vi "Scale Settings Dialog.vi"(8 "error in (no error)":errorcluster, 11 "Scale Module Config In":T1={"GUID"="", "Drop Coords"={"Horizontal"=0, "Vertical"=0}, "Process Name"="", "User name"="", "Queue Name"="", "Settings"={"Cycle Period"=500.0, "Mettler"={"VISA resource name"="", "Simulated?"=FALSE}, "Scale Type"=""}, "Load Count"=0}) -> (0 "error out":errorcluster, 1 "Cancelled?":bool=TRUE, 2 "UI Refresh Needed?":bool, 3 "Scale Module Config Out":T1={"GUID"="", "Drop Coords"={"Horizontal"=0, "Vertical"=0}, "Process Name"="", "User name"="", "Queue Name"="", "Settings"={"Cycle Period"=500.0, "Mettler"={"VISA resource name"="", "Simulated?"=FALSE}, "Scale Type"=""}, "Load Count"=0})   [LabVIEW 2018, in "Scale Module.lvlib"]
doc: "Dialog for selecting user specified settings."
uses:
  Scale Module.lvlib
  Feed Module/Controls/Scale Module Settings Cluster.ctl
  Mettler Toledo/Controls/Settings Cluster.ctl
  Feed Module/Controls/Scale Module Config Cluster.ctl
  <vilib>/Utility/miscctls.llb/LVPoint32TypeDef.ctl
  <vilib>/Utility/xml.llb/Write to XML File(string).vi
  Settings/Settings.lvlib
  Mettler Toledo/Mettler Toledo.lvlib
panel:
  in  "Module Name":string
  in  "Scale Configurations":T3={"Cycle Period"=500.0, "Mettler"={"VISA resource name"="", "Simulated?"=FALSE}, "Scale Type"="Default"}
  in  "Cancel Button":bool
  in  "OK Button":bool
  # "Non visible portion of dialog (needed for connector pane)."
  # "Scale Settings"
  # "Scale Settings"
  # "Scale Settings"
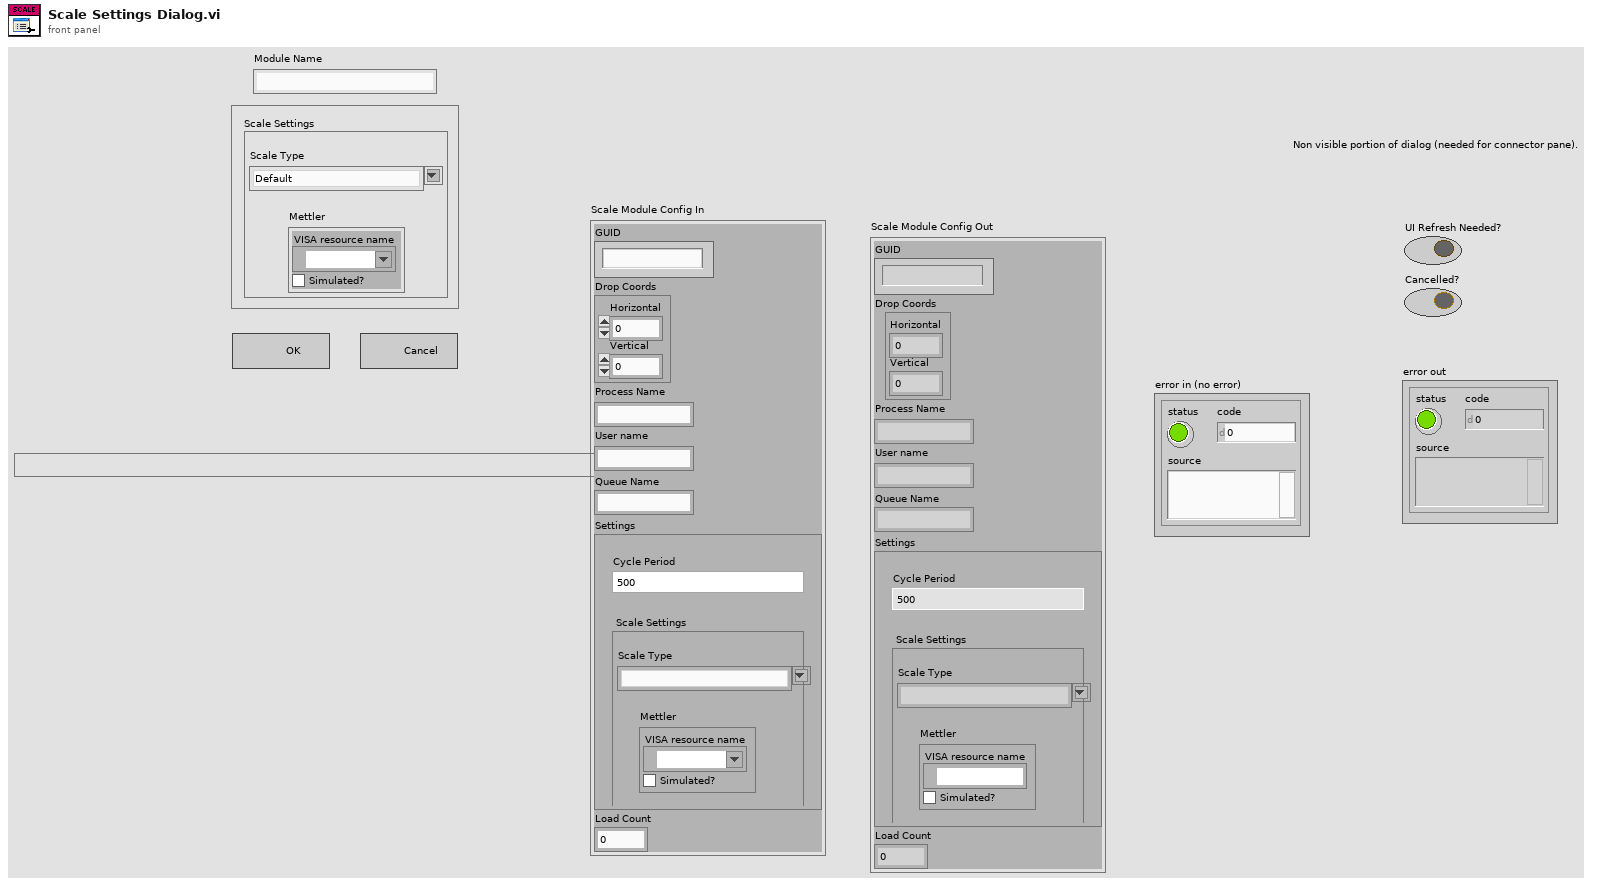
[diagram p1: front panel]
types:
  T1 = typedef "Scale Module.lvlib/Scale Module Config Cluster.ctl" = cluster{"GUID":string, "Drop Coords":T2, "Process Name":string, "User name":string, "Queue Name":string, "Settings":T3, "Load Count":i32}
  T2 = typedef "LVPoint32TypeDef.ctl" = cluster{"Horizontal":i32, "Vertical":i32}
  T3 = typedef "Scale Module.lvlib/Scale Module Settings Cluster.ctl" = cluster{"Cycle Period":dbl, "Mettler":T4, "Scale Type":string}
  T4 = typedef "Mettler Toledo.lvlib/Settings Cluster.ctl" = cluster{"VISA resource name":refnum<visa-resource-name>, "Simulated?":bool}
  T5 = enum8{"Enabled", "Disabled", "Disabled and Grayed Out"}
  T6 = cluster{"Cycle Period":dbl, "Mettler":T4, "Scale Type":string}
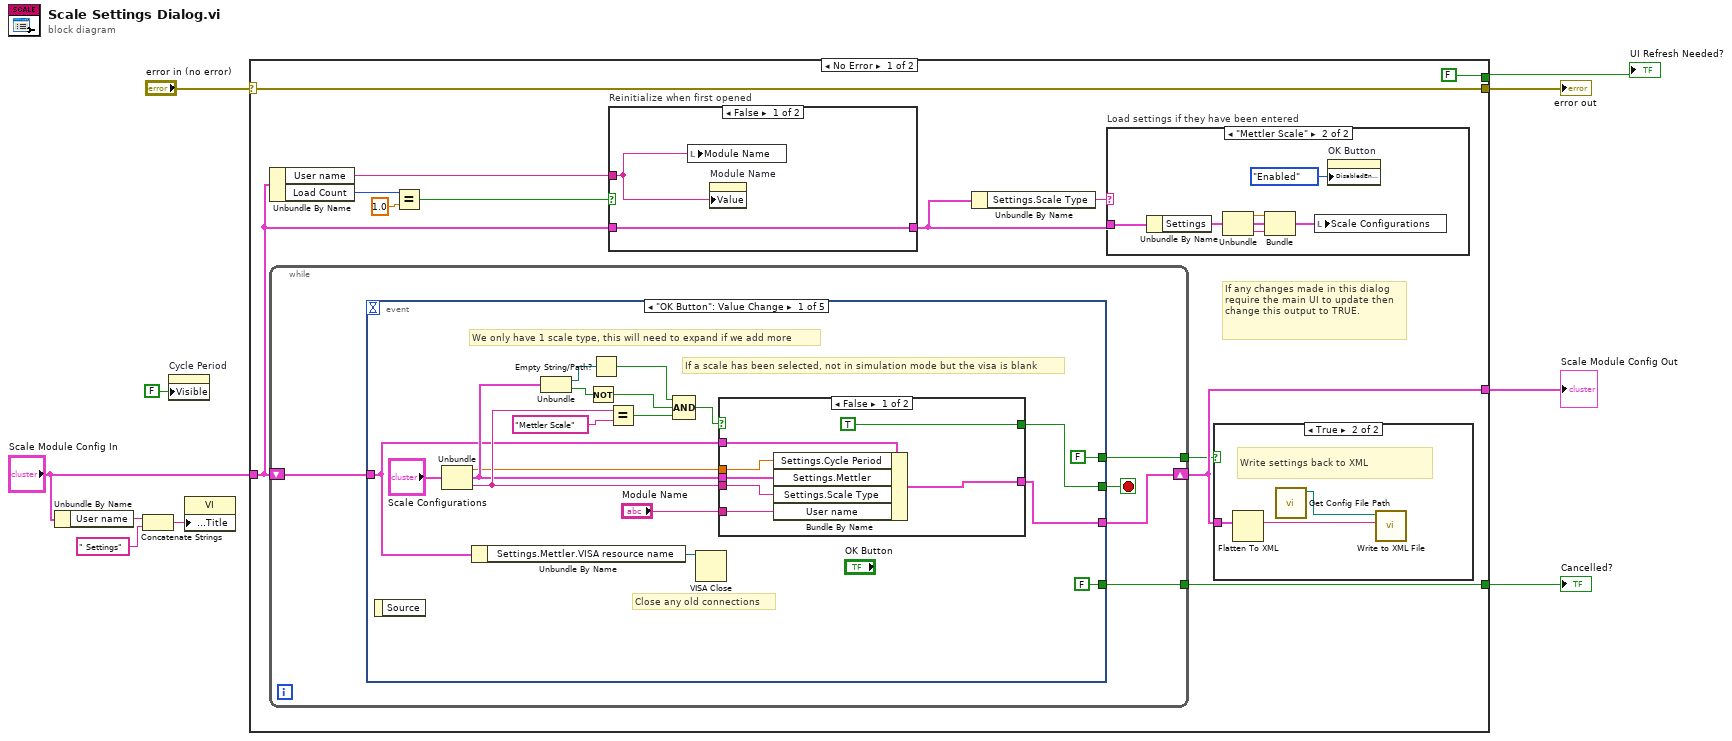
[diagram p0: block diagram]
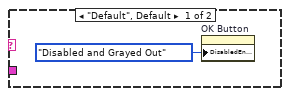
[diagram p2: hidden frame]
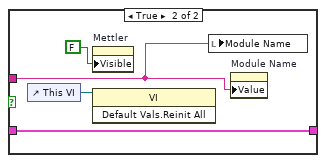
[diagram p3: hidden frame]
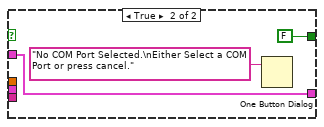
[diagram p4: hidden frame]
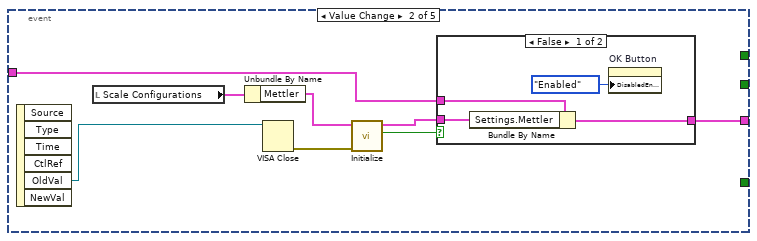
[diagram p5: hidden frame]
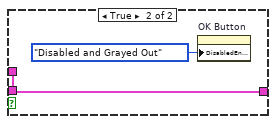
[diagram p6: hidden frame]
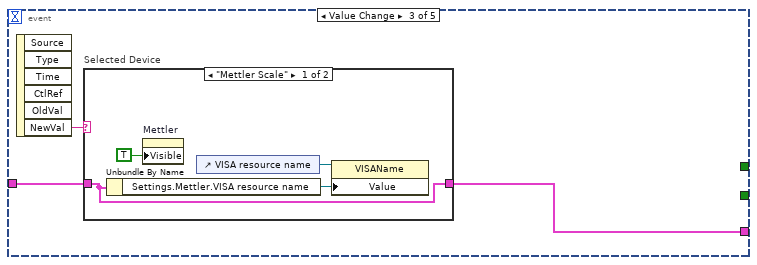
[diagram p7: hidden frame]
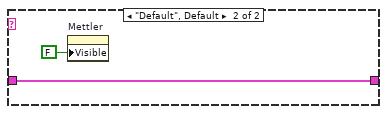
[diagram p8: hidden frame]
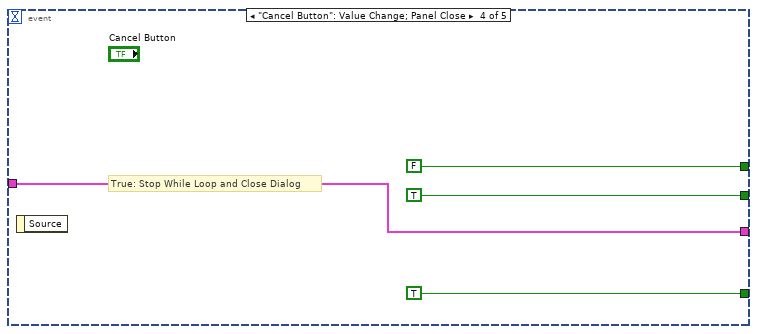
[diagram p9: hidden frame]
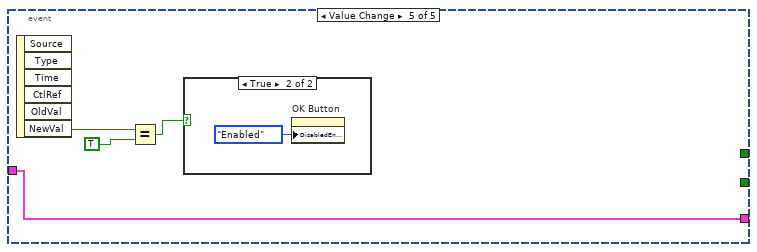
[diagram p10: hidden frame]
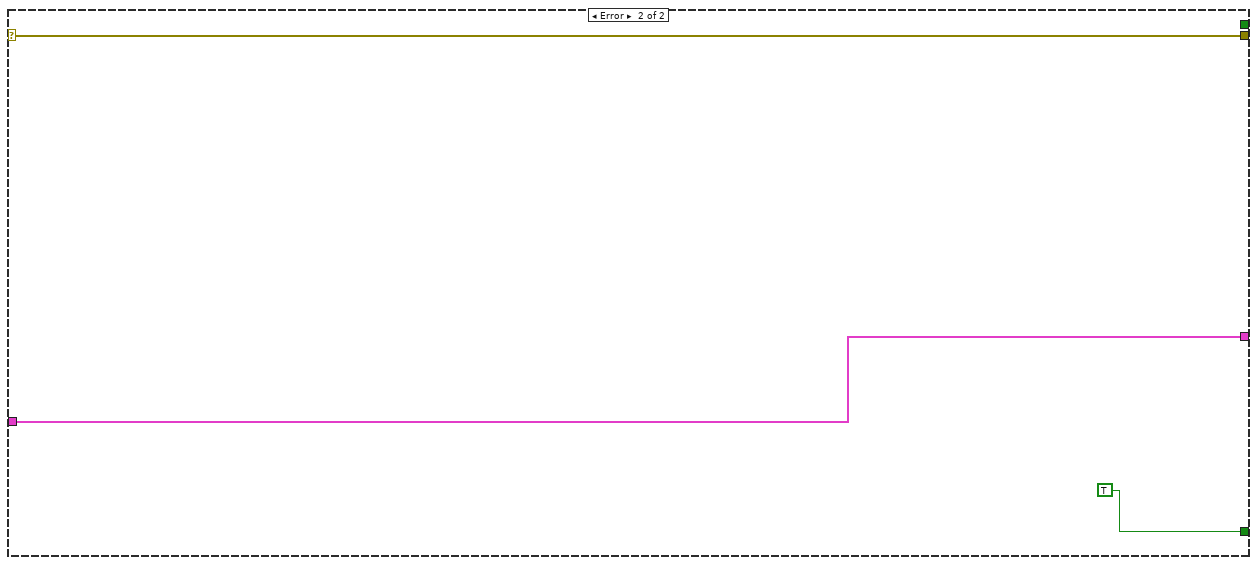
[diagram p13: hidden frame]
diagram:
  n1 = Unbundle By Name("Scale Module Config In") -> ("User name"=w1:string)
  n2 = Concatenate Strings(w1, " Settings" ("string")) -> (w4:string)
  n3 = property on="Cycle Period" class="DigNum (strict)"("Visible"=FALSE) -> ()  [unwired: 2 in, 2 out]
  n4 = property class="VI"("Front Panel.Title"=w4) -> ()  [unwired: 2 in, 2 out]
  n5 = case shown="No Error" "error in (no error)" {
    selector: "error in (no error)" -> [w22 w107]
    tunnel: [w22 w107] -> w10
    tunnel: "Scale Module Config In" -> [w12 w106]
    tunnel: [w20 w106] -> w6
    tunnel: [FALSE ("UI Refresh Needed?") _] -> w9
    tunnel: [w16 TRUE ("UI Refresh Needed?")] -> w8
    frame No Error {
      # "If any changes made in this dialog require the main UI to update then change this output to TRUE."
      n6 = Unbundle By Name(w12) -> ("User name"=w11:string, "Load Count"=w19:i32)
      n7 = while {
        tunnel: [w41] -> w17
        tunnel: [w38] -> w16
        shift-right: [w40] -> w20
        shift-left: w12 -> [w37]
        stop <- w39 stop-if-true
        n8 = event shown="[0] \"OK Button\": Value Change" {
          selector: _ -> [_ _ _ _ _]
          dyn-events: _ -> [_ _ _ _ _]
          timeout: _ -> [_ _ _ _ _]
          tunnel: [w57 w75 w85 w96 w100] -> w40
          tunnel: w37 -> [w48 w76 w84 w96 w100]
          tunnel: [FALSE ("UI Refresh Needed?") _ _ FALSE ("UI Refresh Needed?") _] -> w41
          tunnel: [w58 _ _ TRUE _] -> w39
          tunnel: [FALSE ("UI Refresh Needed?") _ _ TRUE ("UI Refresh Needed?") _] -> w38
          event "OK Button": Value Change {
            # "Close any old connections"
            # "If a scale has been selected, not in simulation mode but the visa is blank"
            # "We only have 1 scale type, this will need to expand if we add more"
            n9 = event-data() -> ()  [unwired: 1 in, 1 out]
            n10 = Unbundle("Scale Configurations") -> ("Cycle Period"=w51:dbl, "Mettler"=w52:T4, "Scale Type"=w54:string)
            n11 = Unbundle By Name(w48) -> ("Settings.Mettler.VISA resource name"=w47:refnum<visa-resource-name>)
            n12 = Unbundle(w52) -> ("VISA resource name"=w55:refnum<visa-resource-name>, "Simulated?"=w50:bool)
            n13 = Not(x=w50) -> (.not. x?=w44:bool)
            n14 = Empty String/Path?(string/path=w55) -> (empty?=w45:bool)
            n15 = Equal?(x=w54, y="Mettler Scale") -> (x = y?=w43:bool)
            n16 = Compound Arithmetic op=AND(w45, w44, w43) -> (w42:bool)
            n17 = VISA Close(VISA resource name=w47) -> ()  [unwired: 1 in, 1 out]
            n18 = case shown="False" w42 {
              tunnel: [TRUE FALSE] -> w58
              tunnel: [w65 w68] -> w57
              tunnel: w48 -> [w64 w68]
              tunnel: w54 -> [w63 _]
              tunnel: w52 -> [w62 _]
              tunnel: w51 -> [w61 _]
              tunnel: "Module Name" -> [w60 _]
              frame False {
                n19 = Bundle By Name(cluster=w64, "Settings.Cycle Period"=w61, "Settings.Mettler"=w62, "Settings.Scale Type"=w63, "User name"=w60) -> (w65:T1)
              }
              frame True {
                n20 = One Button Dialog(message="No COM Port Selected.\nEither Select a COM Port or press cancel.") -> ()  [unwired: 1 in, 1 out]
              }
            }
          }
          event Value Change {
            n21 = event-data() -> ("OldVal"=w71:refnum<visa-resource-name>)  [unwired: 1 in, 5 out]
            n22 = local read "Scale Configurations"() -> (w77:T3)
            n23 = Unbundle By Name(w77) -> ("Mettler"=w74:T4)
            n24 = VISA Close(VISA resource name=w71) -> (error out=w72:errorcluster)  [unwired: 1 in]
            n25 = call "Initialize.vi"("error in (no error)"=w72, "Mettler Settings in"=w74) -> ("No Scale Connected"=w70:bool, "Mettler Settings out"=w73:T4)  [unwired: 7 in, 1 out]
            n26 = case shown="False" w70 {
              tunnel: w76 -> [w81 w83]
              tunnel: [w80 w83] -> w75
              tunnel: w73 -> [w79 _]
              frame False {
                n27 = Bundle By Name(cluster=w81, "Settings.Mettler"=w79) -> (w80:T1)
                n28 = property on="OK Button" class="Bool"("DisabledEnum"=T5."Enabled" ("Disabled")) -> ()  [unwired: 2 in, 2 out]
              }
              frame True {
                n29 = property on="OK Button" class="Bool"("DisabledEnum"=T5."Disabled and Grayed Out" ("Disabled")) -> ()  [unwired: 2 in, 2 out]
              }
            }
          }
          event Value Change {
            n30 = event-data() -> ("NewVal"=w86:string)  [unwired: 1 in, 5 out]
            n31 = case "Selected Device" shown="\"Mettler Scale\"" w86 {
              tunnel: [w87 w92] -> w85
              tunnel: w84 -> [w87 w92]
              frame "Mettler Scale" {
                n32 = Unbundle By Name(w87) -> ("Settings.Mettler.VISA resource name"=w90:refnum<visa-resource-name>)
                n33 = property on="Mettler" class="Clust (strict)"("Visible"=TRUE) -> ()  [unwired: 2 in, 2 out]
                n34 = control-ref of="VISA resource name"() -> (w88:refnum<vi>)
                n35 = property on="Property Node" class="VISAName"(reference=w88, "Value"=w90) -> ()  [unwired: 1 in, 2 out]
              }
              frame "Default", Default {
                n36 = property on="Mettler" class="Clust (strict)"("Visible"=FALSE) -> ()  [unwired: 2 in, 2 out]
              }
            }
          }
          event "Cancel Button": Value Change; Panel Close {
            # "True: Stop While Loop and Close Dialog"
            n37 = event-data() -> ()  [unwired: 1 in, 1 out]
          }
          event Value Change {
            n38 = event-data() -> ("NewVal"=w98:bool)  [unwired: 1 in, 5 out]
            n39 = Equal?(x=w98, y=TRUE) -> (x = y?=w97:bool)
            n40 = case shown="True" w97 {
              frame False {
              }
              frame True {
                n41 = property on="OK Button" class="Bool"("DisabledEnum"=T5."Enabled" ("Disabled")) -> ()  [unwired: 2 in, 2 out]
              }
            }
          }
        }
      }
      n42 = Equal?(x=w19, y=1.0) -> (x = y?=w15:bool)
      n43 = case "Reinitialize when first opened" shown="False" w15 {
        tunnel: w12 -> [w32 w35]
        tunnel: [w32 w35] -> w13
        tunnel: w11 -> [w31 w33]
        frame False {
          n44 = local write "Module Name"(w31) -> ()
          n45 = property on="Module Name" class="Str"("Value"=w31) -> ()  [unwired: 2 in, 2 out]
        }
        frame True {
          n46 = control-ref of="This VI"() -> (w36:refnum<vi>)
          n47 = property on="Mettler" class="Clust (strict)"("Visible"=FALSE) -> ()  [unwired: 2 in, 2 out]
          n48 = invoke class="VI" method="Default Vals.Reinit All"(reference=w36) -> ()  [unwired: 2 in, 3 out]
          n49 = local write "Module Name"(w33) -> ()
          n50 = property on="Module Name" class="Str"("Value"=w33) -> ()  [unwired: 2 in, 2 out]
        }
      }
      n51 = Unbundle By Name(w13) -> ("Settings.Scale Type"=w14:string)
      n52 = case "Load settings if they have been entered" shown="\"Mettler Scale\"" w14 {
        tunnel: w13 -> [_ w25]
        frame "Default", Default {
          n53 = property on="OK Button" class="Bool"("DisabledEnum"=T5."Disabled and Grayed Out" ("Disabled")) -> ()  [unwired: 2 in, 2 out]
        }
        frame "Mettler Scale" {
          n54 = Unbundle By Name(w25) -> ("Settings"=w27:T3)
          n55 = Unbundle(w27) -> ("Cycle Period"=w29:dbl, "Mettler"=w30:T4, "Scale Type"=w26:string)
          n56 = Bundle("Cycle Period"=w29, "Mettler"=w30, "Scale Type"=w26) -> (w28:T6)  [unwired: 1 in]
          n57 = local write "Scale Configurations"(w28) -> ()
          n58 = property on="OK Button" class="Bool"("DisabledEnum"=T5."Enabled" ("Disabled")) -> ()  [unwired: 2 in, 2 out]
        }
      }
      n59 = case shown="True" w17 {
        tunnel: w20 -> [_ w103]
        frame False {
        }
        frame True {
          # "Write settings back to XML"
          n60 = Flatten To XML(anything=w103) -> (xml string=w102:string)
          n61 = call "Get Config File Path.vi"() -> ("XML File Path"=w104:path)  [unwired: 10 in, 1 out]
          n62 = call-poly <vilib>:"Write to XML File.vi"("XML Input"=w102, "XML File Path"=w104) -> ()  [unwired: 7 in, 3 out]
        }
      }
    }
    frame Error {
    }
  }
  "UI Refresh Needed?" <- w9
  "error out" <- w10
  "Cancelled?" <- w8
  "Scale Module Config Out" <- w6
